vi "Offline_Analysis_SWSVM_분석기.vi"(0 "LDA_matrix":path caption="LDA_matrix.txt", 1 "svm_model_file":string, 2 "Group Number":i32, 3 "Target_order.txt":path, 4 "mius_flash_order":path, 5 "Brain":path, 6 "Target":path, 7 "피험자이름":string="홍길동", 8 "Selected":path, 9 "Save_path":string, 10 "Nontarget":path, 11 "W":path, 12 "in_matrix":path caption="in", 13 "전체_Selected":path) -> ()   [LabVIEW 2014]
uses:
  <vilib>/Utility/file.llb/Read From Spreadsheet File (DBL).vi
  <vilib>/Analysis/Matrix/Numeric/Conversions/Array To Matrix - RA2.vi
  <vilib>/Analysis/Matrix/Numeric/Conversions/Array To Matrix - RA.vi
  <vilib>/Utility/file.llb/Read From Spreadsheet File (I64).vi
  <vilib>/Utility/file.llb/Write To Spreadsheet File (DBL).vi
  <vilib>/Utility/file.llb/Write To Spreadsheet File (I64).vi
  <vilib>/Utility/file.llb/Write To Spreadsheet File (string).vi
  <vilib>/Analysis/Matrix/NI_Matrix.lvlib
panel:
  out "ACC":i16
  out "Target_order":i64[](array[numeric])
  out "Selected_Target":i32[](array[numeric])
  out "Accuracy":i16[](array[numeric])
  out "error out":errorcluster
  in  "Random_num":i32=6
  in  "Flash_Repeat":i32=20
  in  "Frame_Length":i32=20
  in  "Sampling_Rate":dbl=512.0
  # "ERP_Parameter안씀. LDA바로 집어넣으면 됨"
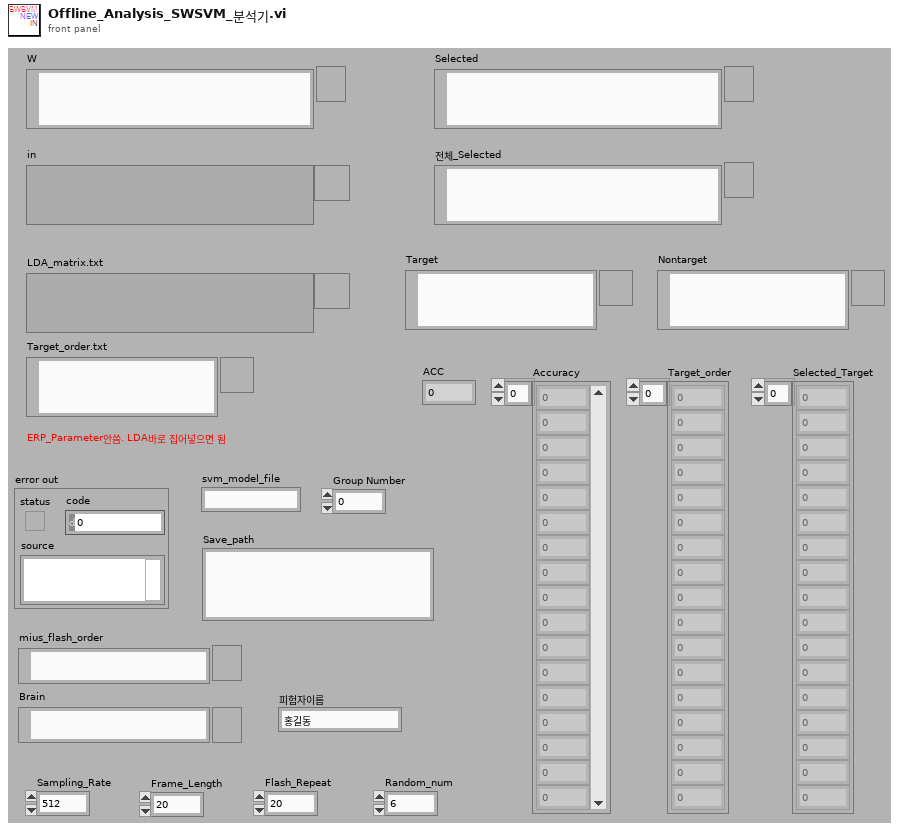
[diagram p1: front panel]
types:
  T1 = typedef "NI_Matrix.lvlib/RealMatrix.ctl" = dbl[][]
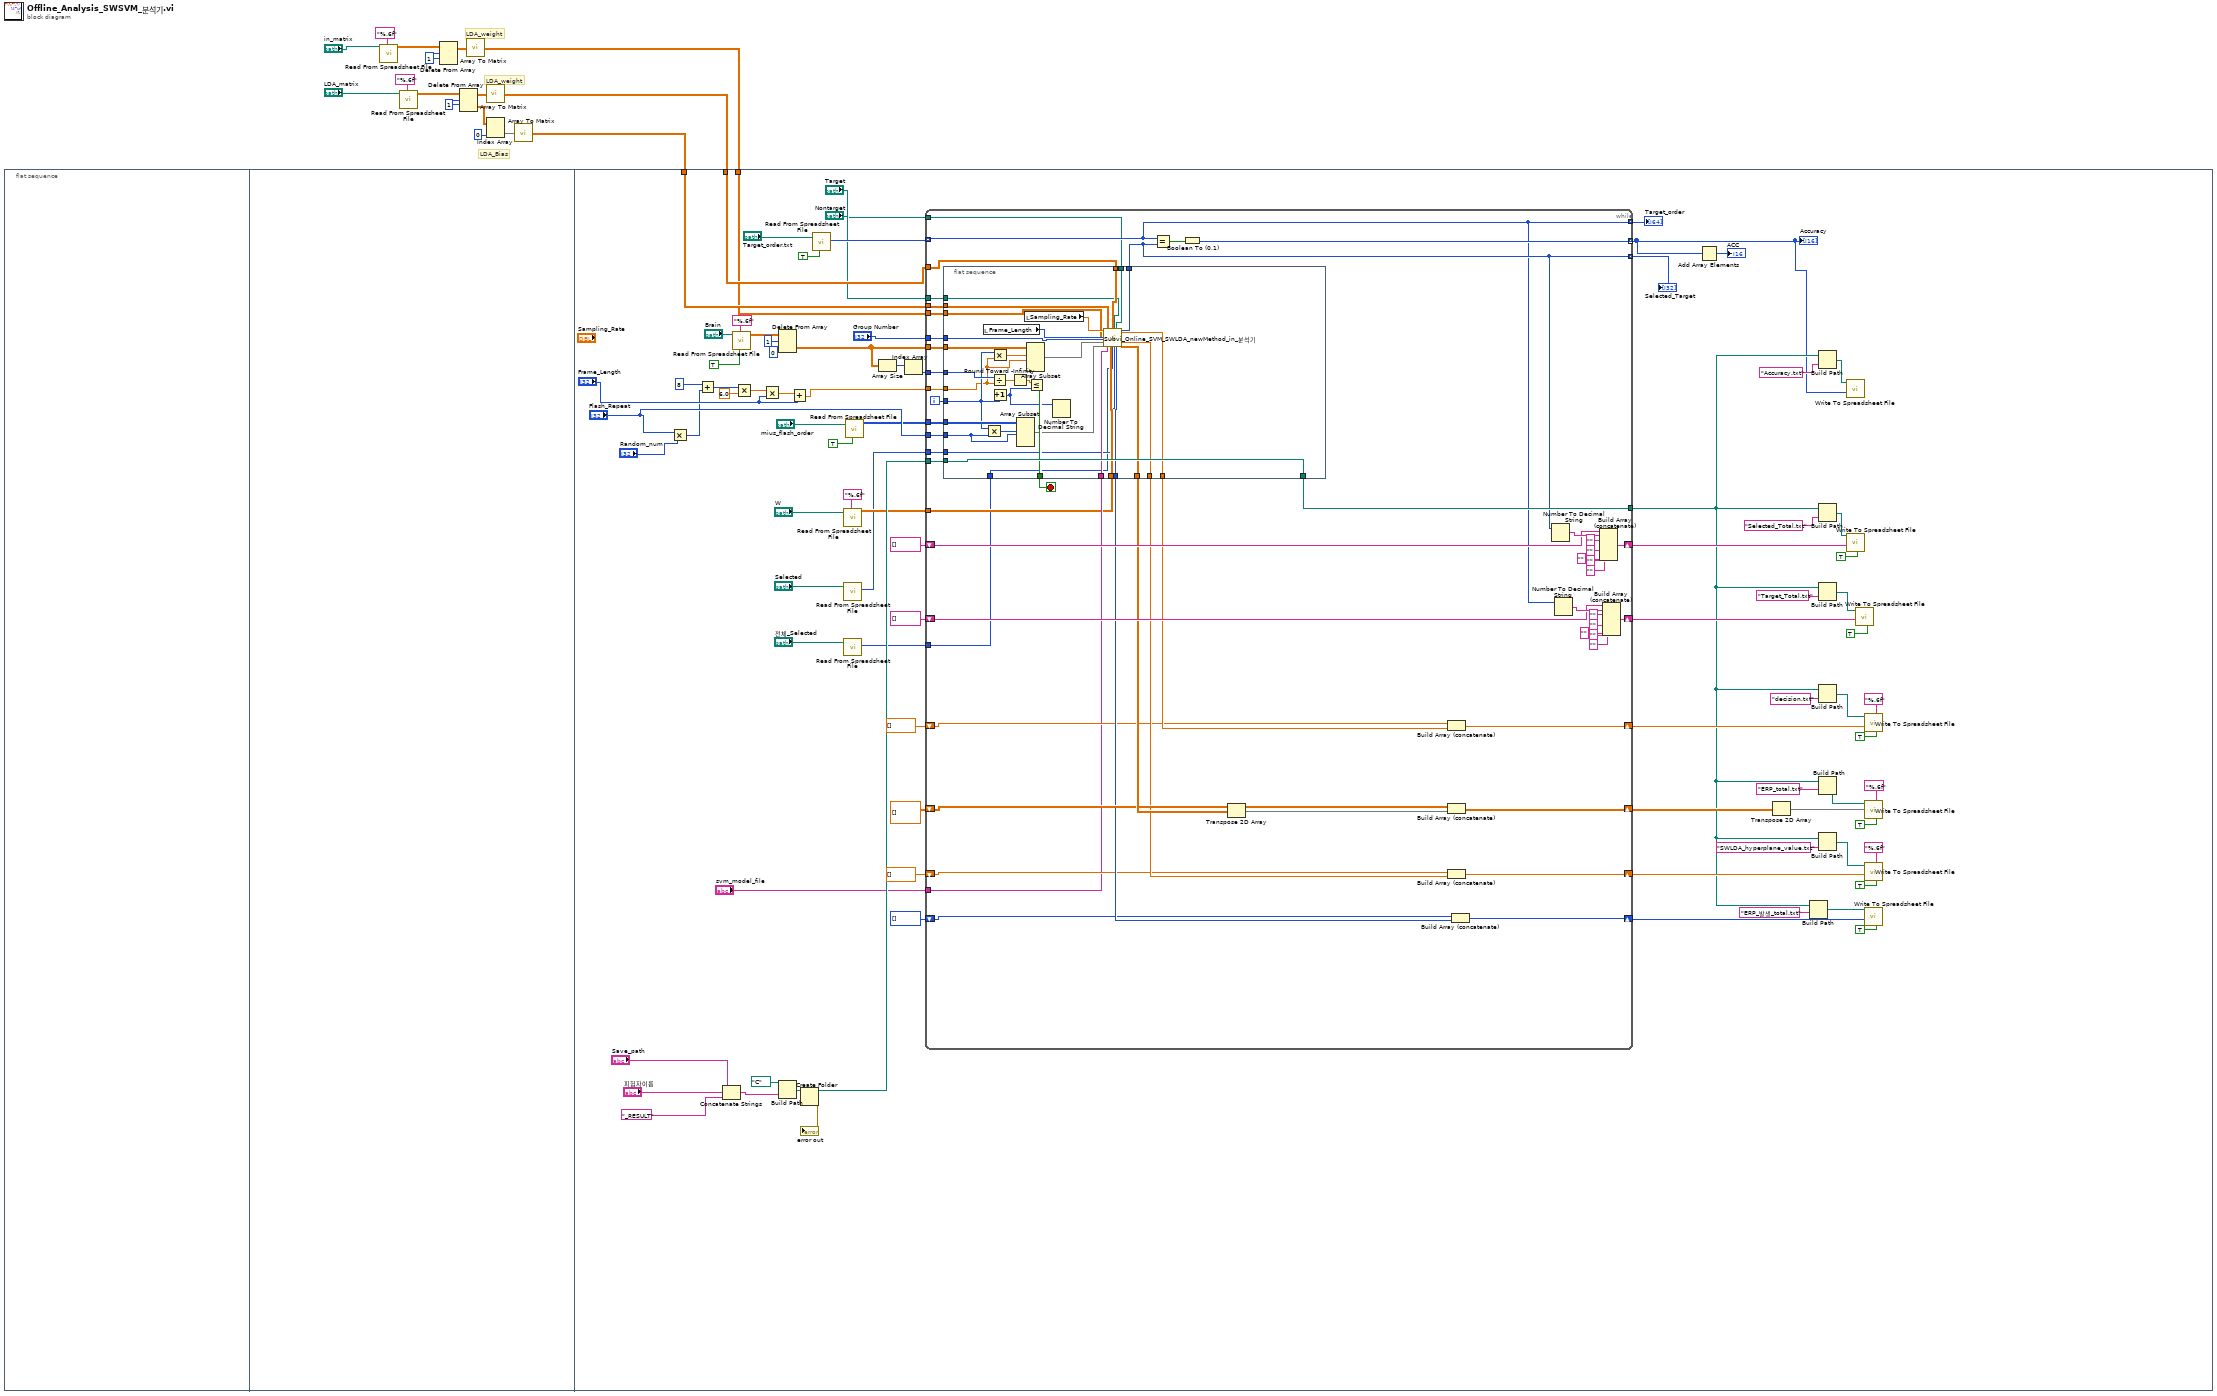
[diagram p0: block diagram]
diagram:
  w4 = 1 ("인덱스 (행)")
  w11 = 1 ("인덱스 (행)")
  # "LDA_weight"
  # "LDA_Bias"
  # "LDA_weight"
  n1 = flat-sequence {
    tunnel: w8 -> [w52]
    tunnel: w7 -> [w51]
    tunnel: w1 -> [w32]
    frame #0 {
    }
    frame #1 {
    }
    frame #2 {
      n2 = Multiply(x="Flash_Repeat", y="Random_num") -> (x*y=w91:i32)
      n3 = Add(x=8, y=w91) -> (x+y=w93:i32)
      n4 = Concatenate Strings("Save_path", "피험자이름", "_RESULT" ("string")) -> (w37:string)
      n5 = call-poly <vilib>:"Read From Spreadsheet File.vi"("transpose (no:F)"=TRUE, "format (%.3f)"="%.6f", "file path (dialog if empty)"="Brain") -> ("all rows"=w85:dbl[][])  [unwired: 4 in, 4 out]
      n6 = Multiply(x=w93, y=6.0) -> (x*y=w95:dbl)
      n7 = Multiply(x=w95, y="Frame_Length") -> (x*y=w97:dbl)
      n8 = Build Path(base path=path "C:/" ("path"), name or relative path=w37) -> (appended path=w100:path)
      n9 = Delete From Array(array=w85, length=1 ("길이"), index (col)=0 ("비활성화된 인덱스 (열)")) -> (deleted portion=w50:dbl[][])  [unwired: 1 in, 1 out]
      n10 = Add(x=w97, y="Frame_Length") -> (x+y=w98:dbl)
      n11 = Create Folder(path (use dialog)=w100) -> (created path=w102:path, error out=→"error out":errorcluster)  [unwired: 2 in, 1 out]
      n12 = call-poly <vilib>:"Read From Spreadsheet File.vi"("transpose (no:F)"=TRUE, "file path (dialog if empty)"="Target_order.txt") -> ("first row"=w79:i64[])  [unwired: 5 in, 4 out]
      n13 = call-poly <vilib>:"Read From Spreadsheet File.vi"("format (%.3f)"="%.6f", "file path (dialog if empty)"="W") -> ("all rows"=w27:dbl[][])  [unwired: 5 in, 4 out]
      n14 = call-poly <vilib>:"Read From Spreadsheet File.vi"("file path (dialog if empty)"="Selected") -> ("first row"=w23:i64[])  [unwired: 6 in, 4 out]
      n15 = call-poly <vilib>:"Read From Spreadsheet File.vi"("file path (dialog if empty)"="전체_Selected") -> ("first row"=w17:i64[])  [unwired: 6 in, 4 out]
      n16 = call-poly <vilib>:"Read From Spreadsheet File.vi"("transpose (no:F)"=TRUE, "file path (dialog if empty)"="mius_flash_order") -> ("all rows"=w87:i64[][])  [unwired: 5 in, 4 out]
      n17 = Array Size(array=w50) -> (size(s)=w88:i32[])
      n18 = Index Array(array=w88) -> (element=w89:i32)  [unwired: 1 in]
      n19 = while {
        tunnel: w51 -> [w156]
        tunnel: w52 -> [w155]
        tunnel: w50 -> [w153]
        tunnel: w87 -> [w152]
        tunnel: w89 -> [w154]
        tunnel: w98 -> [w150]
        tunnel: "Flash_Repeat" -> [w151]
        tunnel: w102 -> [w149]
        tunnel: w79 -> [w128] mode=indexing
        tunnel: [w147] -> w19 mode=indexing
        tunnel: [w128] -> w76 mode=indexing
        tunnel: [w129] -> w77 mode=indexing
        tunnel: [w144] -> w20
        shift-right: [w131] -> w66
        shift-left: string[] [] -> [w130]
        shift-right: [w127] -> w65
        shift-left: string[] [] -> [w126]
        shift-right: [w123] -> w60
        shift-left: dbl[][] [] -> [w122]
        shift-right: [w120] -> w53
        shift-left: i16[] [] -> [w119]
        shift-right: [w117] -> w46
        shift-left: dbl[] [] -> [w116]
        shift-right: [w114] -> w39
        shift-left: dbl[] [] -> [w113]
        tunnel: "svm_model_file" -> [w112]
        tunnel: "Target" -> [w111]
        tunnel: "Nontarget" -> [w110]
        tunnel: w32 -> [w109]
        tunnel: w27 -> [w108]
        tunnel: "Group Number" -> [w107]
        tunnel: w23 -> [w106]
        tunnel: w17 -> [w105]
        i -> [w146]
        stop <- w145 stop-if-true
        n20 = flat-sequence {
          tunnel: [w188] -> w144
          tunnel: w109 -> [w161]
          tunnel: w110 -> [w162]
          tunnel: w111 -> [w163]
          tunnel: w112 -> [w164]
          tunnel: [w165] -> w115
          tunnel: [w166] -> w118
          tunnel: [w168] -> w121
          tunnel: [w169] -> w125
          tunnel: [w170] -> w129
          tunnel: w149 -> [w188]
          tunnel: w150 -> [w176]
          tunnel: w146 -> [w177]
          tunnel: w151 -> [w178]
          tunnel: w152 -> [w180]
          tunnel: w153 -> [w183]
          tunnel: [w184] -> w145
          tunnel: w154 -> [w185]
          tunnel: w155 -> [w186]
          tunnel: w156 -> [w187]
          tunnel: w108 -> [w160]
          tunnel: w107 -> [w159]
          tunnel: w106 -> [w158]
          tunnel: w105 -> [w157]
          frame #0 {
            n21 = local read "Frame_Length"() -> (w172:i32)
            n22 = Multiply(x=w177, y=w178) -> (x*y=w179:i32)
            n23 = Divide(x=w185, y=w176) -> (x/y=w175:dbl)
            n24 = Multiply(x=w177, y=w176) -> (x*y=w182:dbl)
            n25 = Increment(x=w177) -> (x+1=w171:i32)
            n26 = Round Toward -Infinity(1:w175) -> (0:w174:dbl)
            n27 = Array Subset(array=w180, index (row)=w179, length (row)=w178) -> (w167:i64[][])  [unwired: 2 in]
            n28 = local read "Sampling_Rate"() -> (w173:dbl)
            n29 = Array Subset(array=w183, index (row)=w182, length (row)=w176) -> (w181:dbl[][])  [unwired: 2 in]
            n30 = Less Or Equal?(x=w174, y=w171) -> (x <= y?=w184:bool)
            n31 = Number To Decimal String(number=w171) -> ()  [unwired: 1 in, 1 out]
            n32 = call "Subvi_Online_SVM_SWLDA_newMethod_in_분석기.vi"("rate"=w173, "samples per channel"=w172, "in"=w161, "Group Number"=w159, "Brain_data_source"=w181, "Target_Flash_Order"=w167, "Value"=w187, "svm_model_file"=w164, "W"=w160, "Matrix"=w186, "전체_Selected"=w157, "Target"=w163, "Selected"=w158, "Nontarget"=w162) -> ("EPR_발생_total"=w168:i16[], "output-0~8"=w170:i32, "decision"=w165:dbl[], "SWLDA"=w166:dbl[], "ERP_Parameters"=w169:dbl[][])  [unwired: 9 in]
          }
        }
        n33 = Equal?(x=w128, y=w129) -> (x = y?=w148:bool)
        n34 = Boolean To (0,1)(Boolean=w148) -> (0, 1=w147:i16)
        n35 = Transpose 2D Array(2D array=w125) -> (transposed array=w124:dbl[][])
        n36 = Build Array (concatenate)(w113, w115) -> (w114:dbl[])
        n37 = Build Array (concatenate)(w122, w124) -> (w123:dbl[][])
        n38 = Build Array (concatenate)(w116, w118) -> (w117:dbl[])
        n39 = Build Array (concatenate)(w119, w121) -> (w120:i16[])
        n40 = Number To Decimal String(number=w129) -> (decimal integer string=w137:string)  [unwired: 1 in]
        n41 = Number To Decimal String(number=w128) -> (decimal integer string=w143:string)  [unwired: 1 in]
        n42 = Build Array (concatenate)(w130, w137, "" ("element"), "" ("element"), "" ("element"), "" ("element"), "" ("element")) -> (w131:string[])
        n43 = Build Array (concatenate)(w126, w143, "" ("element"), "" ("element"), "" ("element"), "" ("element"), "" ("element")) -> (w127:string[])
      }
      "Accuracy" <- w19
      "Selected_Target" <- w77
      "Target_order" <- w76
      n44 = Add Array Elements(numeric array=w19) -> (sum=→"ACC":i16)
      n45 = Transpose 2D Array(2D array=w60) -> (transposed array=w58:dbl[][])
      n46 = Build Path(base path=w20, name or relative path="ERP_발생_total.txt") -> (appended path=w55:path)
      n47 = Build Path(base path=w20, name or relative path="Accuracy.txt") -> (appended path=w22:path)
      n48 = Build Path(base path=w20, name or relative path="Selected_Total.txt") -> (appended path=w68:path)
      n49 = Build Path(base path=w20, name or relative path="Target_Total.txt") -> (appended path=w73:path)
      n50 = Build Path(base path=w20, name or relative path="decision.txt") -> (appended path=w40:path)
      n51 = Build Path(base path=w20, name or relative path="ERP_total.txt") -> (appended path=w61:path)
      n52 = Build Path(base path=w20, name or relative path="SWLDA_hyperplane_value.txt") -> (appended path=w48:path)
      n53 = call-poly <vilib>:"Write To Spreadsheet File.vi"("1D data"=w19, "file path (dialog if empty)"=w22) -> ()  [unwired: 6 in, 1 out]
      n54 = call-poly <vilib>:"Write To Spreadsheet File.vi"("transpose? (no:F)"=TRUE, "1D data"=w66, "file path (dialog if empty)"=w68) -> ()  [unwired: 5 in, 1 out]
      n55 = call-poly <vilib>:"Write To Spreadsheet File.vi"("transpose? (no:F)"=TRUE, "1D data"=w65, "file path (dialog if empty)"=w73) -> ()  [unwired: 5 in, 1 out]
      n56 = call-poly <vilib>:"Write To Spreadsheet File.vi"("transpose? (no:F)"=TRUE, "format (%.3f)"="%.6f", "1D data"=w39, "file path (dialog if empty)"=w40) -> ()  [unwired: 4 in, 1 out]
      n57 = call-poly <vilib>:"Write To Spreadsheet File.vi"("transpose? (no:F)"=TRUE, "format (%.3f)"="%.6f", "2D data"=w58, "file path (dialog if empty)"=w61) -> ()  [unwired: 4 in, 1 out]
      n58 = call-poly <vilib>:"Write To Spreadsheet File.vi"("transpose? (no:F)"=TRUE, "format (%.3f)"="%.6f", "1D data"=w46, "file path (dialog if empty)"=w48) -> ()  [unwired: 4 in, 1 out]
      n59 = call-poly <vilib>:"Write To Spreadsheet File.vi"("transpose? (no:F)"=TRUE, "1D data"=w53, "file path (dialog if empty)"=w55) -> ()  [unwired: 5 in, 1 out]
    }
  }
  n60 = call-poly <vilib>:"Read From Spreadsheet File.vi"("format (%.3f)"="%.6f", "file path (dialog if empty)"="in_matrix") -> ("all rows"=w3:dbl[][])  [unwired: 5 in, 4 out]
  n61 = call-poly <vilib>:"Read From Spreadsheet File.vi"("format (%.3f)"="%.6f", "file path (dialog if empty)"="LDA_matrix") -> ("all rows"=w9:dbl[][])  [unwired: 5 in, 4 out]
  n62 = Delete From Array(array=w3, length=w4, index (row)=w4) -> (array with subset deleted=w5:dbl[][])  [unwired: 1 in, 1 out]
  n63 = Delete From Array(array=w9, length=w11, index (row)=w11) -> (deleted portion=w14:dbl[][], array with subset deleted=w13:dbl[][])  [unwired: 1 in]
  n64 = call-poly <vilib>:"Array To Matrix.vi"("Real 2D Array"=w5) -> ("Real Matrix"=w1:T1)
  n65 = call-poly <vilib>:"Array To Matrix.vi"("Real 2D Array"=w13) -> ("Real Matrix"=w8:T1)
  n66 = Index Array(array=w14, index (col)=0 ("인덱스")) -> (element=w12:dbl[])  [unwired: 1 in]
  n67 = call-poly <vilib>:"Array To Matrix.vi"("Real 1D Array"=w12) -> ("Real Matrix (Column Vector)"=w7:T1)
